vi "Capture_Image.vi"(7 "New Image":T1, 8 "error in":errorcluster, 10 "ValueDBL":dbl=800000.0, 11 "Session In":T2="cam0") -> (0 "error out":errorcluster, 3 "Image":T1(plugin-control))   [LabVIEW 2011]
uses:
  <vilib>/userdefined/High Color/IMAQdx.ctl
  <vilib>/vision/Image Controls.llb/IMAQ Image.ctl
  <vilib>/vision/driver/NI_Vision_Acquisition_Software.lvlib
  Program Files (x86)/National Instruments/LabVIEW 2011/resource/objmgr/imaqdx.rc
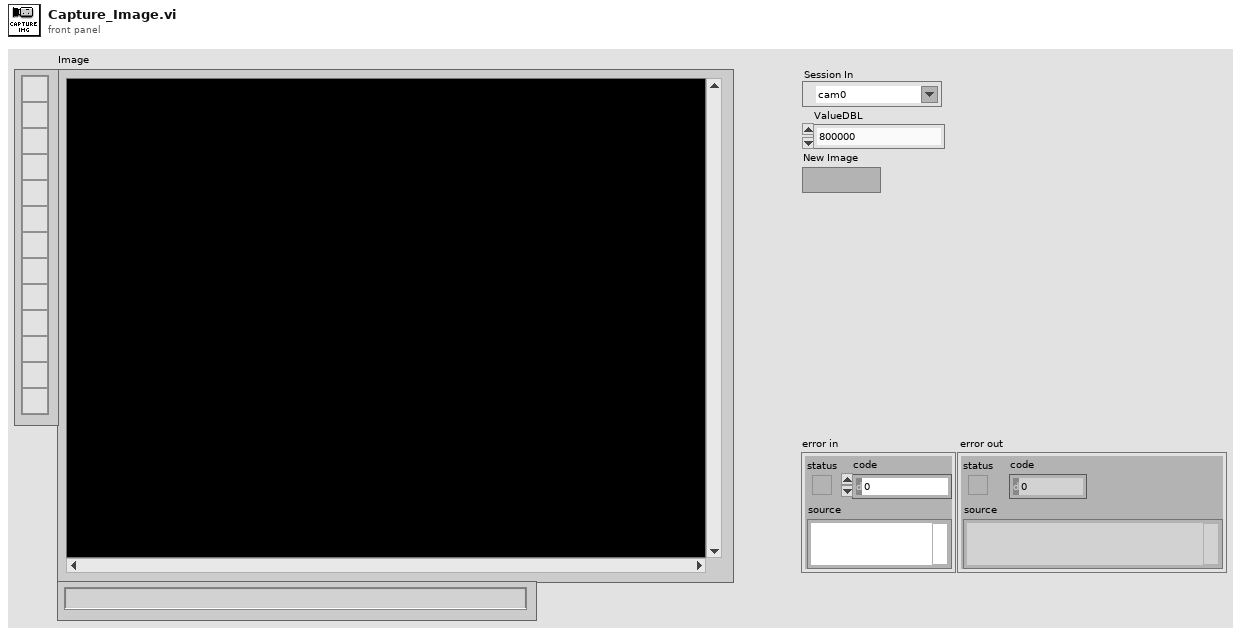
[diagram p1: front panel]
types:
  T1 = typedef "IMAQ Image.ctl" = refnum<image>
  T2 = typedef "IMAQdx.ctl" = refnum<k21>
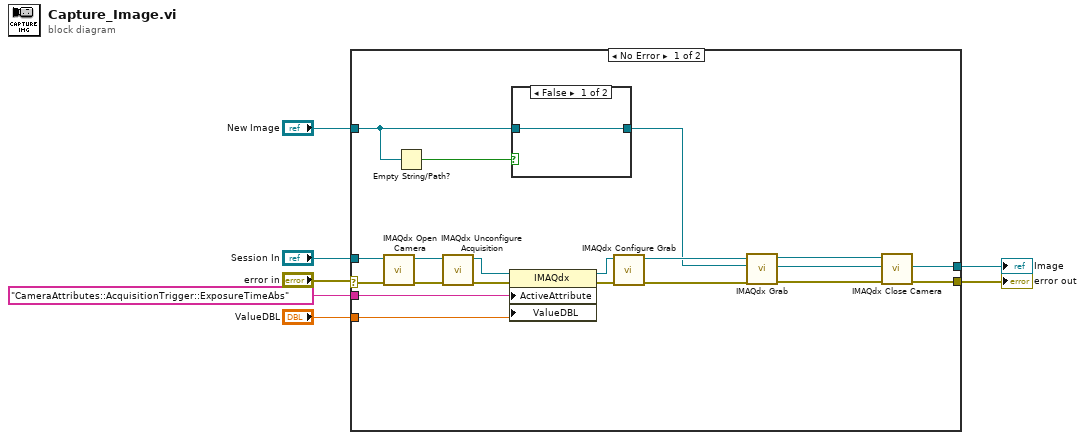
[diagram p0: block diagram]
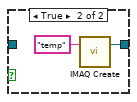
[diagram p2: hidden frame]
diagram:
  n1 = case shown="No Error" "error in" {
    selector: "error in" -> [w10 w30]
    tunnel: "Session In" -> [w26 _]
    tunnel: "CameraAttributes::AcquisitionTrigger::ExposureTimeAbs" ("ActiveAttribute") -> [w21 _]
    tunnel: "ValueDBL" -> [w20 _]
    tunnel: [w12 _] -> w4
    tunnel: [w11 w30] -> w3
    tunnel: "New Image" -> [w8 _]
    frame No Error {
      n2 = call <vilib>:"IMAQdx Open Camera.vi"("error in"=w10, "Session In"=w26) -> ("error out"=w25:errorcluster, "Session Out"=w24:T2)  [unwired: 8 in]
      n3 = Empty String/Path?(string/path=w8) -> (empty?=w9:bool)
      n4 = call <vilib>:"IMAQdx Unconfigure Acquisition.vi"("error in"=w25, "Session In"=w24) -> ("error out"=w23:errorcluster, "Session Out"=w22:T2)  [unwired: 8 in]
      n5 = property class="IMAQdx"(reference=w22, error in=w23, "ActiveAttribute"=w21, "ValueDBL"=w20) -> (reference out=w18:T2, error out=w19:errorcluster)
      n6 = case shown="False" w9 {
        tunnel: [w27 w29] -> w15
        tunnel: w8 -> [w27 _]
        frame False {
        }
        frame True {
          n7 = call "IMAQ Create"("Image Name"="temp") -> ("New Image"=w29:T1)  [unwired: 4 in, 1 out]
        }
      }
      n8 = call <vilib>:"IMAQdx Configure Grab.vi"("error in"=w19, "Session In"=w18) -> ("error out"=w17:errorcluster, "Session Out"=w16:T2)  [unwired: 8 in]
      n9 = call <vilib>:"IMAQdx Grab.vi"("error in"=w17, "Image In"=w15, "Session In"=w16) -> ("error out"=w14:errorcluster, "Image Out"=w12:T1, "Session Out"=w13:T2)  [unwired: 5 in, 1 out]
      n10 = call <vilib>:"IMAQdx Close Camera.vi"("error in"=w14, "Session In"=w13) -> ("error out"=w11:errorcluster)  [unwired: 9 in]
    }
    frame Error {
    }
  }
  "Image" <- w4
  "error out" <- w3
